vi "Convert Boolean string to boolean.vi"(11 "Boolean String":string) -> (3 "Boolean":bool)   [LabVIEW 2015, in "NI_AWS_Core.lvlib"]
uses:
  NI_AWS_Core.lvlib
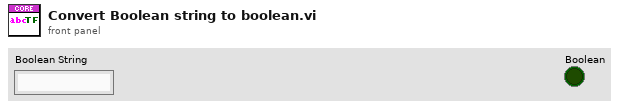
[diagram p1: front panel]
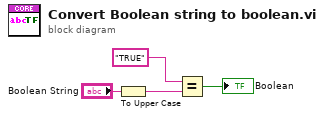
[diagram p0: block diagram]
diagram:
  n1 = To Upper Case(1:"Boolean String") -> (0:w3:string)
  n2 = Equal?(x="TRUE", y=w3) -> (x = y?=→"Boolean":bool)
